vi "SPI Engine. SPI Core.vi"(6 "Ready for Output":bool, 9 "Input Valid":bool, 10 "SPI Information In":T1, 11 "SPI DIO Input":T4) -> (1 "Output Valid":bool, 2 "SPI Output Data":T2, 3 "SPI DIO Output":T3, 4 "Ready For Input":bool, 5 "Chip Select ID":u8)   [LabVIEW 2015]
doc: "This VI performs the actual SPI Transactions. It wraps the SPI Core with added functionality of 4-Wire Handshake"
uses:
  <userlib>/_NI SPI IP/FPGA/Controllers/Public/Spi Master Inputs.ctl
  <userlib>/_NI SPI IP/FPGA/Controllers/Public/Spi Master Outputs.ctl
  Controls/SPI API Response Data.ctl
  Controls/SPI API Transaction Packet.ctl
  <userlib>/_NI SPI IP/FPGA/Controllers/NI SPI IP FPGA.lvlib
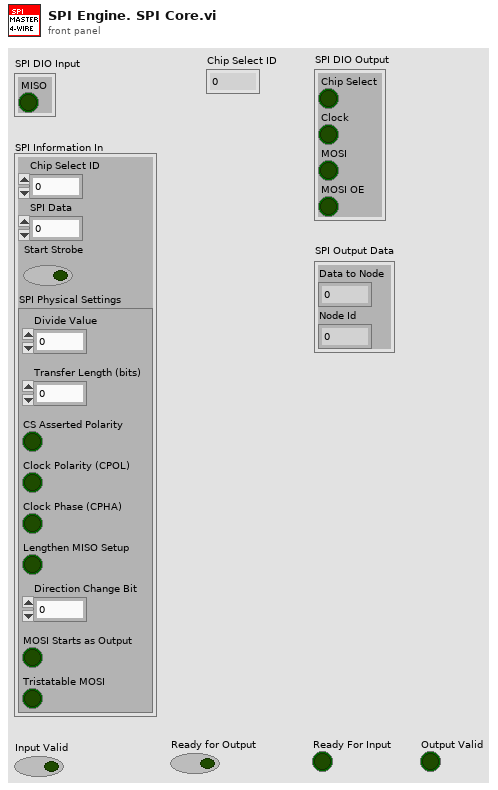
[diagram p1: front panel]
types:
  T1 = typedef "SPI API Transaction Packet.ctl" = cluster{"Chip Select ID":u8, "SPI Data":u64, "Start Strobe":bool, "SPI Physical Settings":cluster{"Divide Value":u8, "Transfer Length (bits)":u8, "CS Asserted Polarity":bool, "Clock Polarity (CPOL)":bool, "Clock Phase (CPHA)":bool, "Lengthen MISO Setup":bool, "Direction Change Bit":u8, "MOSI Starts as Output":bool, "Tristatable MOSI":bool}}
  T2 = typedef "SPI API Response Data.ctl" = cluster{"Data to Node":u64, "Node Id":u16}
  T3 = typedef "NI SPI IP FPGA.lvlib/Spi Master Outputs.ctl" = cluster{"Chip Select":bool, "Clock":bool, "MOSI":bool, "MOSI OE":bool}
  T4 = typedef "NI SPI IP FPGA.lvlib/Spi Master Inputs.ctl" = cluster{"MISO":bool}
  T5 = cluster{"Divide Value":u8, "Transfer Length (bits)":u8, "CS Asserted Polarity":bool, "Clock Polarity (CPOL)":bool, "Clock Phase (CPHA)":bool, "Lengthen MISO Setup":bool, "Direction Change Bit":u8, "MOSI Starts as Output":bool, "Tristatable MOSI":bool}
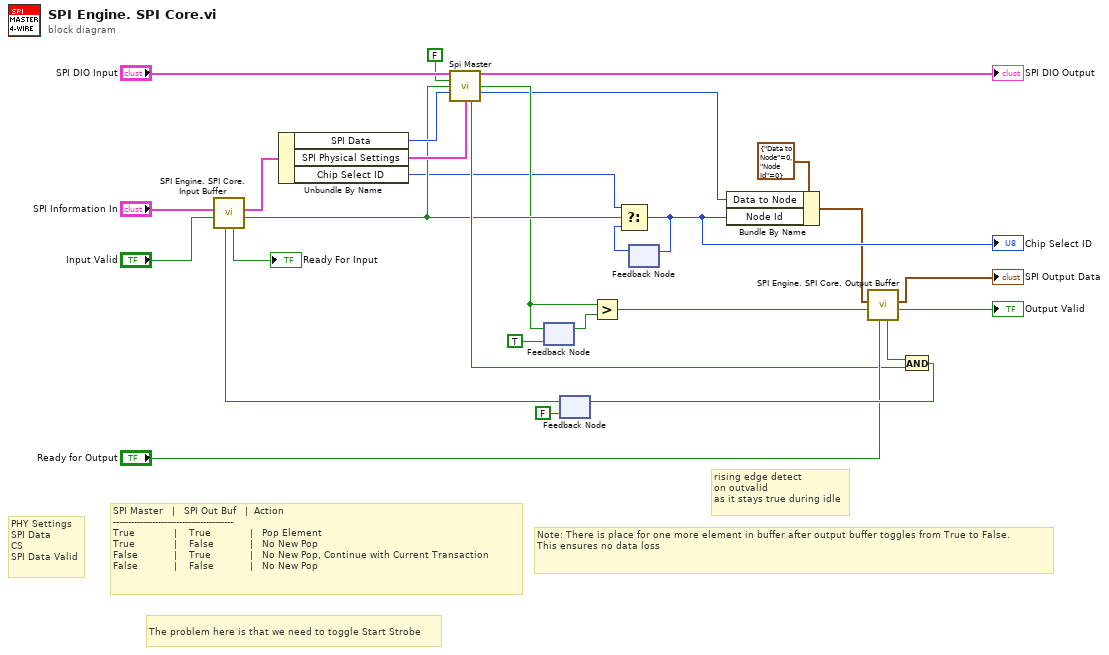
[diagram p0: block diagram]
diagram:
  # "rising edge detect\non outvalid\nas it stays true during idle"
  # "PHY Settings\nSPI Data\nCS\nSPI Data Valid"
  # "The problem here is that we need to toggle Start Strobe"
  # "Note: There is place for one more element in buffer after output buffer toggles from True to False.\nThis ensures no data loss"
  # "SPI Master   |   SPI Out Buf   |  Action\n----------------------------------------\nTrue             |    True             |   Pop Element\nTrue             |    False            |   No New Pop \nFalse            |    True             |   No New Pop, Continue with Current Transaction\nFalse            |    False            |   No New Pop"
  n1 = feedback #1(TRUE ("read data valid")) -> (w11:bool)
  n2 = feedback #2(FALSE) -> (w26:bool)
  n3 = call "SPI Engine. SPI Core. Input Buffer.vi"("Ready for Output"=w26, "Input Valid"="Input Valid", "SPI Information In"="SPI Information In") -> ("Output Valid"=w6:bool, "SPI Information Out"=w8:T1, "Ready For Input"=→"Ready For Input":bool)  [unwired: 6 in]
  n4 = Unbundle By Name(w8) -> ("SPI Data"=w7:u64, "SPI Physical Settings"=w20:T5, "Chip Select ID"=w2:u8)
  n5 = call <userlib>:"Spi Master.vi"("spi input"="SPI DIO Input", "manual assert chip select"=FALSE, "start strobe"=w6, "data to write"=w7, "spi transfer settings"=w20) -> ("spi output"=→"SPI DIO Output":T3, "read data valid"=w4:bool, "read data"=w3:u64, "ready for input"=w10:bool)  [unwired: 7 in]
  n6 = feedback-in #1(w4) -> ()
  n7 = Greater?(x=w4, y=w11) -> (0:w12:bool)
  n8 = feedback #3() -> (w15:u8)  [unwired: 1 in]
  n9 = Select(t=w2, s=w6, f=w15) -> (s? t:f=w5:u8)
  "Chip Select ID" <- w5
  n10 = feedback-in #3(w5) -> ()
  n11 = Bundle By Name(cluster=T2 {"Data to Node"=0, "Node Id"=0} ("SPI Response"), "Data to Node"=w3, "Node Id"=w5) -> (w1:T2)
  n12 = call "SPI Engine. SPI Core. Output Buffer.vi"("Ready for Output"="Ready for Output", "Input Valid"=w12, "Input Data"=w1) -> ("Output Valid"=→"Output Valid":bool, "Output Data"=→"SPI Output Data":T2, "Ready For Input"=w28:bool)  [unwired: 6 in]
  n13 = And(x=w28, y=w10) -> (x .and. y?=w27:bool)
  n14 = feedback-in #2(w27) -> ()
